vi "stop async worker.vi"(8 "error in":errorcluster, 9 "timeout (500 ms)":u16, 10 "run flag in":u8 format="%.0b", 11 "module data in":T1={"run state"=enum."sync", "module"=refnum, "module ref"=refnum, "async exec ref"={"command fifo"=refnum, "error fifo"=refnum, "VI Refnum"=refnum, "input buffer"=refnum, "output buffer"=refnum, "process buffer"=refnum, "original dvrs"=[]}, "configuration ref"=refnum, "GUID"={"Hi"=0, "Lo"=0}, "error"={"status"=FALSE, "code"=0, "source"=""}, "previous error code"=0, "input method"={"data table"={"Double"=[], "Single"=[], "I64"=[], "I32"=[], "I16"=[], "I8"=[], "U64"=[], "U32"=[], "U16"=[], "U8"=[], "Boolean"=[], "String"=[], "Array of Double"=[], "Array of Single"=[], "Array of I64"=[], "Array of I32"=[], "Array of I16"=[], "Array of I8"=[], "Array of U64"=[], "Array of U32"=[], "Array of U16"=[], "Array of U8"=[], "Array of Boolean"=[], "Array of String"=[]}, "transfer spec"=[]}, "output method"={"data table"={"Double"=[], "Single"=[], "I64"=[], "I32"=[], "I16"=[], "I8"=[], "U64"=[], "U32"=[], "U16"=[], "U8"=[], "Boolean"=[], "String"=[], "Array of Double"=[], "Array of Single"=[], "Array of I64"=[], "Array of I32"=[], "Array of I16"=[], "Array of I8"=[], "Array of U64"=[], "Array of U32"=[], "Array of U16"=[], "Array of U8"=[], "Array of Boolean"=[], "Array of String"=[]}, "transfer spec"=[]}, "process method parameters"={"data table"={"Double"=[], "Single"=[], "I64"=[], "I32"=[], "I16"=[], "I8"=[], "U64"=[], "U32"=[], "U16"=[], "U8"=[], "Boolean"=[], "String"=[], "Array of Double"=[], "Array of Single"=[], "Array of I64"=[], "Array of I32"=[], "Array of I16"=[], "Array of I8"=[], "Array of U64"=[], "Array of U32"=[], "Array of U16"=[], "Array of U8"=[], "Array of Boolean"=[], "Array of String"=[]}, "transfer spec"=[]}, "process method results"={"data table"={"Double"=[], "Single"=[], "I64"=[], "I32"=[], "I16"=[], "I8"=[], "U64"=[], "U32"=[], "U16"=[], "U8"=[], "Boolean"=[], "String"=[], "Array of Double"=[], "Array of Single"=[], "Array of I64"=[], "Array of I32"=[], "Array of I16"=[], "Array of I8"=[], "Array of U64"=[], "Array of U32"=[], "Array of U16"=[], "Array of U8"=[], "Array of Boolean"=[], "Array of String"=[]}, "transfer spec"=[]}, "fault handling"={"unknown"=[], "trivial"=[], "critical"=[], "recoverable"=[]}, "error report index "=-1} {"GUID"."Lo" format="%.0x"; "GUID"."Hi" format="%.0x"}) -> (0 "error out":errorcluster, 2 "run flag out":u8 format="%.0b", 3 "module data out":T1={"run state"=enum."sync", "module"=refnum, "module ref"=refnum, "async exec ref"={"command fifo"=refnum, "error fifo"=refnum, "VI Refnum"=refnum, "input buffer"=refnum, "output buffer"=refnum, "process buffer"=refnum, "original dvrs"=[]}, "configuration ref"=refnum, "GUID"={"Hi"=0, "Lo"=0}, "error"={"status"=FALSE, "code"=0, "source"=""}, "previous error code"=0, "input method"={"data table"={"Double"=[], "Single"=[], "I64"=[], "I32"=[], "I16"=[], "I8"=[], "U64"=[], "U32"=[], "U16"=[], "U8"=[], "Boolean"=[], "String"=[], "Array of Double"=[], "Array of Single"=[], "Array of I64"=[], "Array of I32"=[], "Array of I16"=[], "Array of I8"=[], "Array of U64"=[], "Array of U32"=[], "Array of U16"=[], "Array of U8"=[], "Array of Boolean"=[], "Array of String"=[]}, "transfer spec"=[]}, "output method"={"data table"={"Double"=[], "Single"=[], "I64"=[], "I32"=[], "I16"=[], "I8"=[], "U64"=[], "U32"=[], "U16"=[], "U8"=[], "Boolean"=[], "String"=[], "Array of Double"=[], "Array of Single"=[], "Array of I64"=[], "Array of I32"=[], "Array of I16"=[], "Array of I8"=[], "Array of U64"=[], "Array of U32"=[], "Array of U16"=[], "Array of U8"=[], "Array of Boolean"=[], "Array of String"=[]}, "transfer spec"=[]}, "process method parameters"={"data table"={"Double"=[], "Single"=[], "I64"=[], "I32"=[], "I16"=[], "I8"=[], "U64"=[], "U32"=[], "U16"=[], "U8"=[], "Boolean"=[], "String"=[], "Array of Double"=[], "Array of Single"=[], "Array of I64"=[], "Array of I32"=[], "Array of I16"=[], "Array of I8"=[], "Array of U64"=[], "Array of U32"=[], "Array of U16"=[], "Array of U8"=[], "Array of Boolean"=[], "Array of String"=[]}, "transfer spec"=[]}, "process method results"={"data table"={"Double"=[], "Single"=[], "I64"=[], "I32"=[], "I16"=[], "I8"=[], "U64"=[], "U32"=[], "U16"=[], "U8"=[], "Boolean"=[], "String"=[], "Array of Double"=[], "Array of Single"=[], "Array of I64"=[], "Array of I32"=[], "Array of I16"=[], "Array of I8"=[], "Array of U64"=[], "Array of U32"=[], "Array of U16"=[], "Array of U8"=[], "Array of Boolean"=[], "Array of String"=[]}, "transfer spec"=[]}, "fault handling"={"unknown"=[], "trivial"=[], "critical"=[], "recoverable"=[]}, "error report index "=-1} {"GUID"."Lo" format="%.0x"; "GUID"."Hi" format="%.0x"})   [LabVIEW 2013, in "async executor.lvlib"]
uses:
  async executor.lvlib
  Runtime/full module data.ctl
  <vilib>/NI/Tag Bus Module Framework/runtime/TBM module execution interface.lvclass
  Runtime/module run state.ctl
  asynchronous executor reference.ctl
  message to executor.ctl
  Runtime/async command notification.ctl
  <vilib>/NI/Tag Bus/table/data table.ctl
  Runtime/async error info.ctl
  <vilib>/NI/Tag Bus Module Framework/runtime/error classification.ctl
  <vilib>/NI/Tag Bus Module Framework/module configuration/TBM module configuration.lvclass
  <vilib>/NI/Configuration Framework/serializable configuration/Numeric GUID.ctl
  Runtime/module method data.ctl
  <vilib>/NI/Tag Bus/table/transfer specification.ctl
  <vilib>/NI/Tag Bus/tag/Data Type.ctl
  Runtime/fault handling spec.ctl
  Configuration/Error Actions.ctl
  main engine/main engine.lvlib
  <vilib>/NI/Tag Bus/table/data table.lvlib
  <vilib>/NI/Configuration Framework/serializable configuration/NISE_CEF_serializable configuration.lvclass
  <vilib>/NI/Tag Bus/tag/tag descriptor.lvclass
  Configuration/Standard Engine Configuration.lvclass
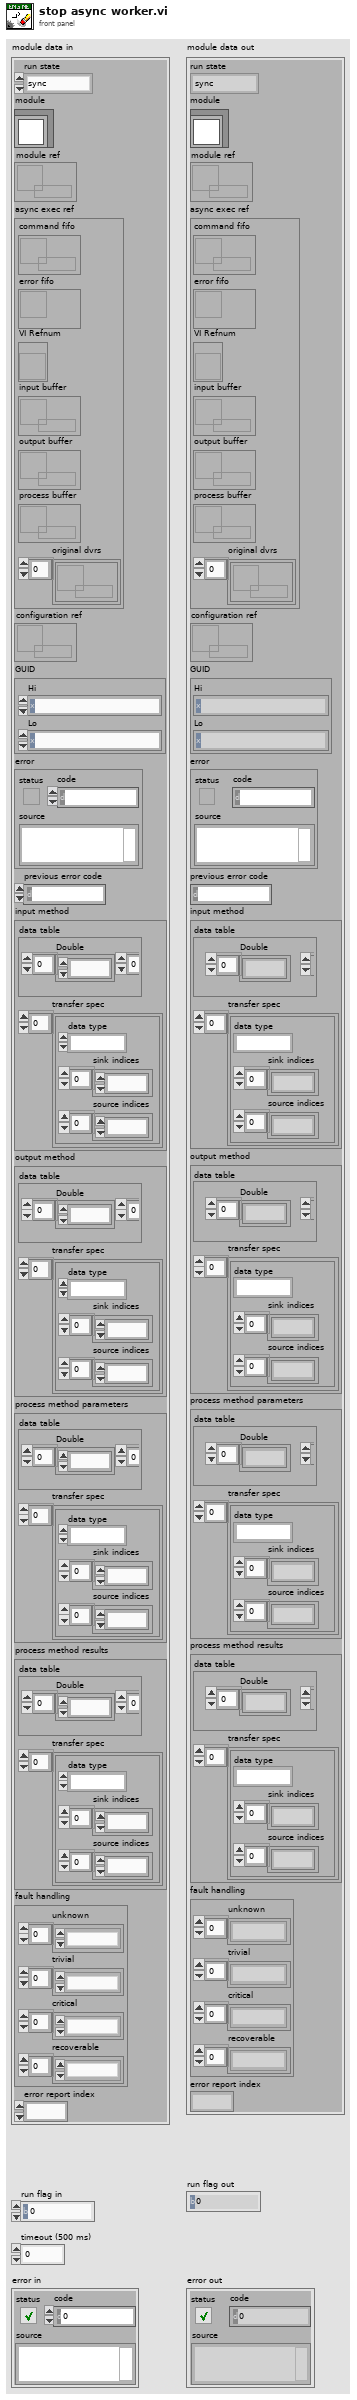
[diagram p1: front panel]
types:
  T1 = typedef "main engine.lvlib/full module data.ctl" = cluster{"run state":T2, "module":refnum<class "TBM module execution interface.lvclass">, "module ref":refnum<data-value>, "async exec ref":T3, "configuration ref":refnum<data-value>, "GUID":T4, "error":errorcluster, "previous error code":i32, "input method":T5, "output method":T5, "process method parameters":T5, "process method results":T5, "fault handling":T9, "error report index ":i32}
  T2 = typedef "main engine.lvlib/module run state.ctl" = enum16{"sync", "async"}
  T3 = typedef "async executor.lvlib/asynchronous executor reference.ctl" = cluster{"command fifo":refnum<k33>, "error fifo":refnum<k33>, "VI Refnum":refnum<vi>, "input buffer":refnum<k33>, "output buffer":refnum<k33>, "process buffer":refnum<k33>, "original dvrs":refnum<data-value>[]}
  T4 = typedef "NISE_CEF_serializable configuration.lvclass/Numeric GUID.ctl" = cluster{"Hi":u64, "Lo":u64}
  T5 = typedef "main engine.lvlib/module method data.ctl" = cluster{"data table":T6, "transfer spec":T7[]}
  T6 = typedef "tag bus.lvlib/data table.lvlib/data table.ctl" = cluster{"Double":dbl[], "Single":sgl[], "I64":i64[], "I32":i32[], "I16":i16[], "I8":i8[], "U64":u64[], "U32":u32[], "U16":u16[], "U8":u8[], "Boolean":bool[], "String":string[], "Array of Double":cluster{"DBL Array":dbl[]}[], "Array of Single":cluster{"SGL Array":sgl[]}[], "Array of I64":cluster{"I64 Array":i64[]}[], "Array of I32":cluster{"I32 Array":i32[]}[], "Array of I16":cluster{"I16 Array":i16[]}[], "Array of I8":cluster{"I8 Array":i8[]}[], "Array of U64":cluster{"U64 Array":u64[]}[], "Array of U32":cluster{"U32 Array":u32[]}[], "Array of U16":cluster{"U16 Array":u16[]}[], "Array of U8":cluster{"U8 Array":u8[]}[], "Array of Boolean":cluster{"Boolean Array":bool[]}[], "Array of String":cluster{"String Array":string[]}[]}
  T7 = typedef "tag bus.lvlib/data table.lvlib/transfer specification.ctl" = cluster{"data type":T8, "sink indices":i32[], "source indices":i32[]}
  T8 = typedef "tag bus.lvlib/tag descriptor.lvclass/Data Type.ctl" = enum16{"Double", "Single", "I64", "I32", "I16", "I8", "U64", "U32", "U16", "U8", "Boolean", "String", "Array of Double", "Array of Single", "Array of I64", "Array of I32", "Array of I16", "Array of I8", "Array of U64", "Array of U32", "Array of U16", "Array of U8", "Array of Boolean", "Array of String"}
  T9 = typedef "main engine.lvlib/fault handling spec.ctl" = cluster{"unknown":T10[], "trivial":T10[], "critical":T10[], "recoverable":T10[]}
  T10 = typedef "Standard Engine Configuration.lvclass/Error Actions.ctl" = enum16{"Clear", "Notify", "Stop Component", "Stop Engine", "Safe State", "Attempt Recovery"}
  T11 = typedef "async executor.lvlib/async command notification.ctl" = enum16{"stop", "input", "process", "output"}
  T12 = typedef "async executor.lvlib/message to executor.ctl" = cluster{"command":T11, "data 1 (i,o,pp)":refnum<data-value>, "data 2 (pr)":refnum<data-value>, "user value":u64}
  T13 = enum32{"Bad", "Idle", "Run top level", "Running"}
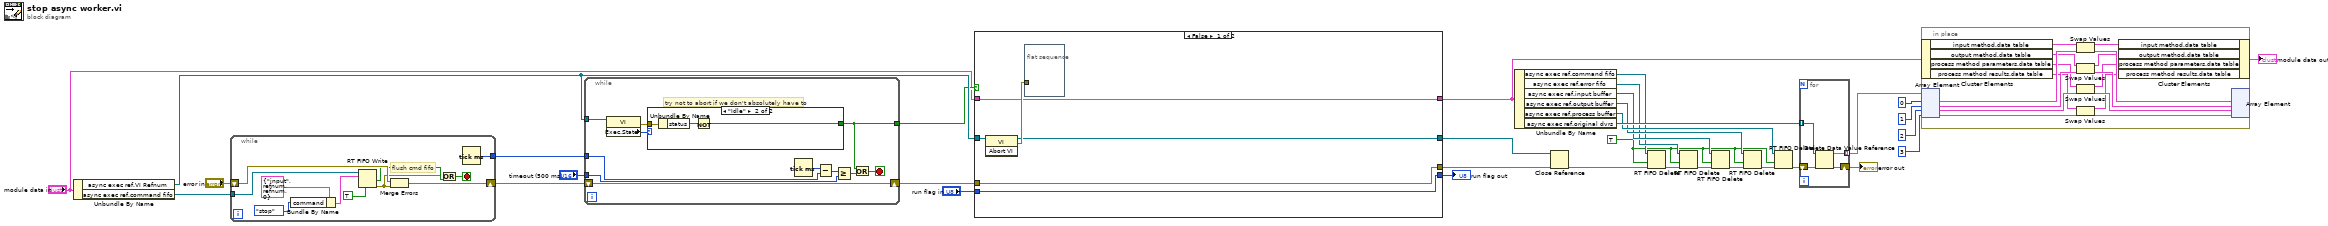
[diagram p0: block diagram]
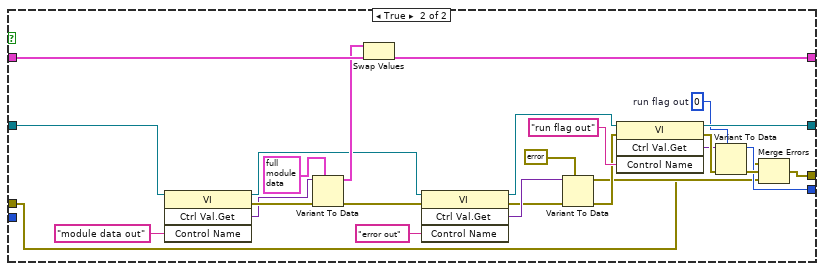
[diagram p2: hidden frame]
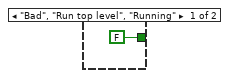
[diagram p3: hidden frame]
diagram:
  w9 = TRUE ("force destroy? (F)")
  n1 = Unbundle By Name("module data in") -> ("async exec ref.VI Refnum"=w29:refnum<vi>, "async exec ref.command fifo"=w31:refnum<k33>)
  n2 = while {
    tunnel: w31 -> [w45]
    shift-right: [w43] -> w34
    shift-left: "error in" -> [w42]
    tunnel: [w38] -> w33
    stop <- w40 stop-if-true
    # "flush cmd fifo"
    n3 = Bundle By Name(cluster=T12 {"command"=enum."input", "data 1 (i,o,pp)"=refnum, "data 2 (pr)"=refnum, "user value"=0} ("element"), "command"=async_command_notification."stop") -> (w36:T12)
    n4 = RT FIFO Write(0:w45, 1:w36, 5:TRUE ("overwrite on timeout (T)")) -> (10:w41:bool, 11:w39:errorcluster)  [unwired: 2 in, 2 out]
    n5 = Merge Errors(w42, w39) -> (w43:errorcluster)
    n6 = Or(x=w39, y=w41) -> (x .or. y?=w40:bool)
    n7 = Tick Count (ms)() -> (millisecond timer value=w38:u32)
  }
  n8 = while {
    shift-right: [w49] -> w28
    shift-left: w34 -> [w49]
    tunnel: w33 -> [w54]
    tunnel: "timeout (500 ms)" -> [w52]
    tunnel: w29 -> [w56]
    tunnel: [w46] -> w27
    stop <- w50 stop-if-true
    # "try not to abort if we don't absolutely have to"
    n9 = property class="VI"(reference=w56) -> (error out=w48:errorcluster, "Exec.State"=w47:T13)  [unwired: 1 in, 1 out]
    n10 = case shown="\"Idle\"" w47 {
      tunnel: w48 -> [_ w60]
      tunnel: [FALSE ("status") w58] -> w46
      frame "Bad", "Run top level", "Running" {
      }
      frame "Idle" {
        n11 = Unbundle By Name(w60) -> ("status"=w59:bool)
        n12 = Not(x=w59) -> (.not. x?=w58:bool)
      }
    }
    n13 = Tick Count (ms)() -> (millisecond timer value=w55:u32)
    n14 = Subtract(x=w55, y=w54) -> (x-y=w53:u32)
    n15 = Greater Or Equal?(x=w53, y=w52) -> (x >= y?=w51:bool)
    n16 = Or(x=w46, y=w51) -> (x .or. y?=w50:bool)
  }
  n17 = case shown="False" w27 {
    tunnel: w29 -> [w66 w88]
    tunnel: w28 -> [w61 w67]
    tunnel: "module data in" -> [w64 w87]
    tunnel: [w64 w85] -> w7
    tunnel: "run flag in" -> [w63 _]
    tunnel: [w63 w71] -> w24
    tunnel: [w62 w73] -> w23
    tunnel: [w61 w69] -> w22
    frame False {
      n18 = invoke class="VI" method="Abort VI"(reference=w66) -> (reference out=w62:refnum<vi>, error out=w65:errorcluster)  [unwired: 2 in, 1 out]
      n19 = flat-sequence {
        tunnel: w65 -> [_]
        frame #0 {
        }
      }
    }
    frame True {
      w72 = u8 0  # run flag out
      n20 = invoke class="VI" method="Ctrl Val.Get"(reference=w88, "Control Name"="module data out") -> (reference out=w76:refnum<vi>, error out=w91:errorcluster, "Get Control Value Variant"=w90:variant)  [unwired: 2 in, 1 out]
      n21 = Variant To Data(error in=w91, type=T1 {"run state"=enum."sync", "module"=refnum, "module ref"=refnum, "async exec ref"={"command fifo"=refnum, "error fifo"=refnum, "VI Refnum"=refnum, "input buffer"=refnum, "output buffer"=refnum, "process buffer"=refnum, "original dvrs"=[]}, "configuration ref"=refnum, "GUID"={"Hi"=0, "Lo"=0}, "error"={"status"=FALSE, "code"=0, "source"=""}, "previous error code"=0, "input method"={"data table"={"Double"=[], "Single"=[], "I64"=[], "I32"=[], "I16"=[], "I8"=[], "U64"=[], "U32"=[], "U16"=[], "U8"=[], "Boolean"=[], "String"=[], "Array of Double"=[], "Array of Single"=[], "Array of I64"=[], "Array of I32"=[], "Array of I16"=[], "Array of I8"=[], "Array of U64"=[], "Array of U32"=[], "Array of U16"=[], "Array of U8"=[], "Array of Boolean"=[], "Array of String"=[]}, "transfer spec"=[]}, "output method"={"data table"={"Double"=[], "Single"=[], "I64"=[], "I32"=[], "I16"=[], "I8"=[], "U64"=[], "U32"=[], "U16"=[], "U8"=[], "Boolean"=[], "String"=[], "Array of Double"=[], "Array of Single"=[], "Array of I64"=[], "Array of I32"=[], "Array of I16"=[], "Array of I8"=[], "Array of U64"=[], "Array of U32"=[], "Array of U16"=[], "Array of U8"=[], "Array of Boolean"=[], "Array of String"=[]}, "transfer spec"=[]}, "process method parameters"={"data table"={"Double"=[], "Single"=[], "I64"=[], "I32"=[], "I16"=[], "I8"=[], "U64"=[], "U32"=[], "U16"=[], "U8"=[], "Boolean"=[], "String"=[], "Array of Double"=[], "Array of Single"=[], "Array of I64"=[], "Array of I32"=[], "Array of I16"=[], "Array of I8"=[], "Array of U64"=[], "Array of U32"=[], "Array of U16"=[], "Array of U8"=[], "Array of Boolean"=[], "Array of String"=[]}, "transfer spec"=[]}, "process method results"={"data table"={"Double"=[], "Single"=[], "I64"=[], "I32"=[], "I16"=[], "I8"=[], "U64"=[], "U32"=[], "U16"=[], "U8"=[], "Boolean"=[], "String"=[], "Array of Double"=[], "Array of Single"=[], "Array of I64"=[], "Array of I32"=[], "Array of I16"=[], "Array of I8"=[], "Array of U64"=[], "Array of U32"=[], "Array of U16"=[], "Array of U8"=[], "Array of Boolean"=[], "Array of String"=[]}, "transfer spec"=[]}, "fault handling"={"unknown"=[], "trivial"=[], "critical"=[], "recoverable"=[]}, "error report index "=-1} ("module data in"), Variant=w90) -> (data=w86:T1, error out=w77:errorcluster)
      n22 = Swap Values(12:w86, 14:w87) -> (3:w85:T1)  [unwired: 1 in, 1 out]
      n23 = invoke class="VI" method="Ctrl Val.Get"(reference=w76, error in=w77, "Control Name"="error out") -> (reference out=w75:refnum<vi>, error out=w83:errorcluster, "Get Control Value Variant"=w84:variant)  [unwired: 1 in, 1 out]
      n24 = Variant To Data(error in=w83, type=errorcluster {"status"=FALSE, "code"=0, "source"=""} ("error constant"), Variant=w84) -> (data=w68:errorcluster, error out=w78:errorcluster)
      n25 = invoke class="VI" method="Ctrl Val.Get"(reference=w75, error in=w78, "Control Name"="run flag out") -> (reference out=w73:refnum<vi>, error out=w80:errorcluster, "Get Control Value Variant"=w79:variant)  [unwired: 1 in, 1 out]
      n26 = Variant To Data(error in=w80, type=w72, Variant=w79) -> (data=w71:u8, error out=w74:errorcluster)
      n27 = Merge Errors(w67, w74, w68) -> (w69:errorcluster)
    }
  }
  "run flag out" <- w24
  n28 = Unbundle By Name(w7) -> ("async exec ref.command fifo"=w10:refnum<k33>, "async exec ref.error fifo"=w11:refnum<k33>, "async exec ref.input buffer"=w12:refnum<k33>, "async exec ref.output buffer"=w13:refnum<k33>, "async exec ref.process buffer"=w14:refnum<k33>, "async exec ref.original dvrs"=w19:refnum<data-value>[])
  n29 = Close Reference(reference=w23, error in (no error)=w22) -> (error out=w21:errorcluster)
  n30 = RT FIFO Delete(0:w10, 2:w9, 3:w21) -> (11:w18:errorcluster)
  n31 = RT FIFO Delete(0:w11, 2:w9, 3:w18) -> (11:w17:errorcluster)
  n32 = RT FIFO Delete(0:w12, 2:w9, 3:w17) -> (11:w16:errorcluster)
  n33 = RT FIFO Delete(0:w13, 2:w9, 3:w16) -> (11:w15:errorcluster)
  n34 = RT FIFO Delete(0:w14, 2:w9, 3:w15) -> (11:w8:errorcluster)
  n35 = for {
    tunnel: w19 -> [w94] mode=indexing
    shift-right: [w95] -> w20
    shift-left: w8 -> [w96]
    tunnel: [w93] -> w5 mode=indexing
    n36 = Delete Data Value Reference(data value reference=w94, error in=w96) -> (data value=w93:T6, error out=w95:errorcluster)
  }
  "error out" <- w20
  n37 = in-place {
    n38 = in-place-cluster #1(w7) -> ("input method.data table"=w104:T6, "output method.data table"=w101:T6, "process method parameters.data table"=w100:T6, "process method results.data table"=w97:T6)
    n39 = in-place-array #2(w5, 0, 1, 2, 3) -> (w105:T6, w108:T6, w109:T6, w112:T6)
    n40 = Swap Values(12:w104, 14:w105) -> (1:w103:T6, 3:w106:T6)  [unwired: 1 in]
    n41 = Swap Values(12:w101, 14:w108) -> (1:w102:T6, 3:w107:T6)  [unwired: 1 in]
    n42 = Swap Values(12:w100, 14:w109) -> (1:w99:T6, 3:w110:T6)  [unwired: 1 in]
    n43 = Swap Values(12:w97, 14:w112) -> (1:w98:T6, 3:w111:T6)  [unwired: 1 in]
    n44 = in-place-cluster #1("input method.data table"=w103, "output method.data table"=w102, "process method parameters.data table"=w99, "process method results.data table"=w98) -> (→"module data out":T1)
    n45 = in-place-array #2(w106, w107, w110, w111) -> ()  [unwired: 5 out]
  }
